vi "Position String.vi"(11 "Reframed Position (m)":cluster{"x (m)":dbl, "y (m)":dbl, "z (m)":dbl} {"z (m)" format="%.1p"; "y (m)" format="%.1p"; "x (m)" format="%.1p"}) -> ()   [LabVIEW 2019]
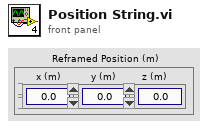
[diagram p1: front panel]
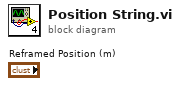
[diagram p0: block diagram]
diagram:
